vi "PDUS-SerialPortDataParse.vi"(9 "Numeric":i32, 10 "ErrorIntput":errorcluster, 11 "InputStr":string) -> (2 "ErrorOutput":errorcluster, 3 "OutputStr":string)   [LabVIEW 2023]
panel:
  out "TempNum":dbl=10.5556
  out "PressNum":dbl=10.5556
  out "Str":string
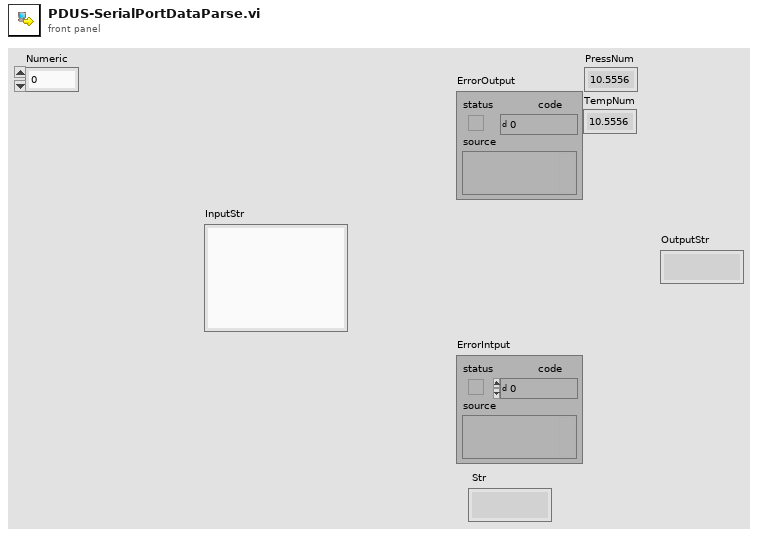
[diagram p1: front panel]
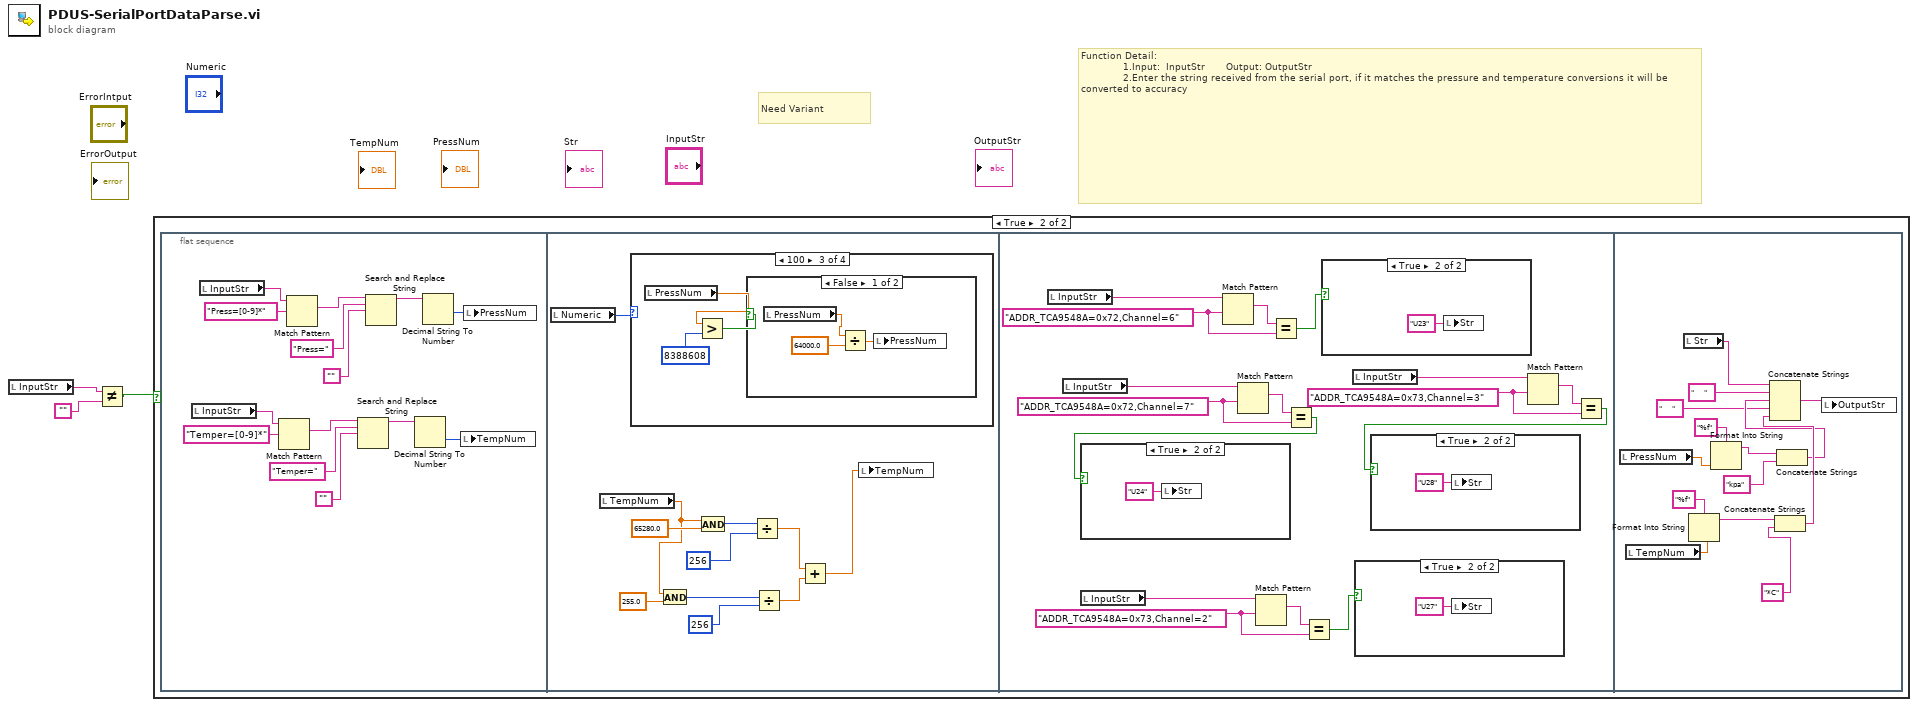
[diagram p0: block diagram]
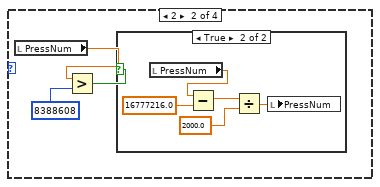
[diagram p4: hidden frame]
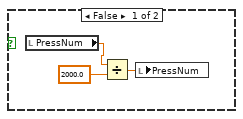
[diagram p5: hidden frame]
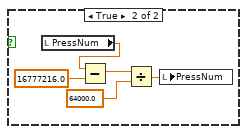
[diagram p6: hidden frame]
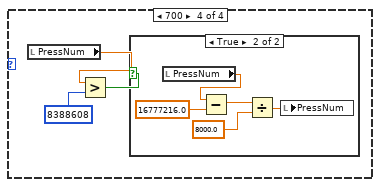
[diagram p7: hidden frame]
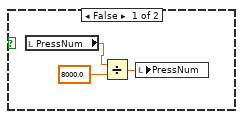
[diagram p8: hidden frame]
diagram:
  # "Function Detail:\n              1.Input:  InputStr       Output: OutputStr\n              2.Enter the string received from the serial port, if it matches the pressure and temperature conversions it will be converted to accuracy"
  # "Need Variant"
  n1 = local read "InputStr"() -> (w3:string)
  n2 = Not Equal?(x=w3, y="") -> (x != y?=w1:bool)
  n3 = case shown="True" w1 {
    frame False {
    }
    frame True {
      n4 = flat-sequence {
        frame #0 {
          n5 = local read "InputStr"() -> (w7:string)
          n6 = local read "InputStr"() -> (w16:string)
          n7 = Match Pattern(string=w7, regular expression="Temper=[0-9]*") -> (match substring=w8:string)  [unwired: 1 in, 3 out]
          n8 = Match Pattern(string=w16, regular expression="Press=[0-9]*") -> (match substring=w15:string)  [unwired: 1 in, 3 out]
          n9 = Search and Replace String(input string=w8, search string="Temper=", replace string="") -> (result string=w11:string)  [unwired: 5 in, 3 out]
          n10 = Search and Replace String(input string=w15, search string="Press=", replace string="") -> (result string=w12:string)  [unwired: 5 in, 3 out]
          n11 = Decimal String To Number(string=w11) -> (number=w4:i32)  [unwired: 2 in, 1 out]
          n12 = Decimal String To Number(string=w12) -> (number=w5:i32)  [unwired: 2 in, 1 out]
          n13 = local write "TempNum"(w4) -> ()
          n14 = local write "PressNum"(w5) -> ()
        }
        frame #1 {
          n15 = local read "Numeric"() -> (w28:i32)
          n16 = local read "TempNum"() -> (w22:dbl)
          n17 = case shown="100" w28 {
            frame 0, Default {
            }
            frame 2 {
              n18 = local read "PressNum"() -> (w30:dbl)
              n19 = Greater?(x=w30, y=8388608) -> (0:w31:bool)
              n20 = case shown="True" w31 {
                frame False {
                  n21 = local read "PressNum"() -> (w33:dbl)
                  n22 = Divide(x=w33, y=2000.0) -> (x/y=w34:dbl)
                  n23 = local write "PressNum"(w34) -> ()
                }
                frame True {
                  n24 = local read "PressNum"() -> (w39:dbl)
                  n25 = Subtract(x=w39, y=16777216.0) -> (x-y=w37:dbl)
                  n26 = Divide(x=w37, y=2000.0) -> (x/y=w35:dbl)
                  n27 = local write "PressNum"(w35) -> ()
                }
              }
            }
            frame 100 {
              n28 = local read "PressNum"() -> (w41:dbl)
              n29 = Greater?(x=w41, y=8388608) -> (0:w42:bool)
              n30 = case shown="False" w42 {
                frame False {
                  n31 = local read "PressNum"() -> (w44:dbl)
                  n32 = Divide(x=w44, y=64000.0) -> (x/y=w45:dbl)
                  n33 = local write "PressNum"(w45) -> ()
                }
                frame True {
                  n34 = local read "PressNum"() -> (w50:dbl)
                  n35 = Subtract(x=w50, y=16777216.0) -> (x-y=w48:dbl)
                  n36 = Divide(x=w48, y=64000.0) -> (x/y=w46:dbl)
                  n37 = local write "PressNum"(w46) -> ()
                }
              }
            }
            frame 700 {
              n38 = local read "PressNum"() -> (w52:dbl)
              n39 = Greater?(x=w52, y=8388608) -> (0:w53:bool)
              n40 = case shown="True" w53 {
                frame False {
                  n41 = local read "PressNum"() -> (w55:dbl)
                  n42 = Divide(x=w55, y=8000.0) -> (x/y=w56:dbl)
                  n43 = local write "PressNum"(w56) -> ()
                }
                frame True {
                  n44 = local read "PressNum"() -> (w61:dbl)
                  n45 = Subtract(x=w61, y=16777216.0) -> (x-y=w59:dbl)
                  n46 = Divide(x=w59, y=8000.0) -> (x/y=w57:dbl)
                  n47 = local write "PressNum"(w57) -> ()
                }
              }
            }
          }
          n48 = And(x=w22, y=255.0) -> (x .and. y?=w23:i32)
          n49 = And(x=w22, y=65280.0) -> (x .and. y?=w26:i32)
          n50 = Divide(x=w26, y=256) -> (x/y=w20:dbl)
          n51 = Divide(x=w23, y=256) -> (x/y=w19:dbl)
          n52 = Add(x=w20, y=w19) -> (x+y=w18:dbl)
          n53 = local write "TempNum"(w18) -> ()
        }
        frame #2 {
          w64 = "ADDR_TCA9548A=0x73,Channel=2" ("regular expression")
          w66 = "ADDR_TCA9548A=0x73,Channel=3" ("regular expression")
          w73 = "ADDR_TCA9548A=0x72,Channel=7" ("regular expression")
          w75 = "ADDR_TCA9548A=0x72,Channel=6" ("regular expression")
          n54 = local read "InputStr"() -> (w77:string)
          n55 = local read "InputStr"() -> (w71:string)
          n56 = local read "InputStr"() -> (w62:string)
          n57 = Match Pattern(string=w77, regular expression=w75) -> (match substring=w76:string)  [unwired: 1 in, 3 out]
          n58 = Match Pattern(string=w71, regular expression=w73) -> (match substring=w72:string)  [unwired: 1 in, 3 out]
          n59 = Match Pattern(string=w62, regular expression=w64) -> (match substring=w63:string)  [unwired: 1 in, 3 out]
          n60 = Equal?(x=w76, y=w75) -> (x = y?=w74:bool)
          n61 = Equal?(x=w72, y=w73) -> (x = y?=w70:bool)
          n62 = case shown="True" w70 {
            frame False {
            }
            frame True {
              n63 = local write "Str"("U24" ("Str")) -> ()
            }
          }
          n64 = Equal?(x=w63, y=w64) -> (x = y?=w65:bool)
          n65 = case shown="True" w74 {
            frame False {
            }
            frame True {
              n66 = local write "Str"("U23" ("Str")) -> ()
            }
          }
          n67 = local read "InputStr"() -> (w68:string)
          n68 = case shown="True" w65 {
            frame False {
            }
            frame True {
              n69 = local write "Str"("U27" ("Str")) -> ()
            }
          }
          n70 = Match Pattern(string=w68, regular expression=w66) -> (match substring=w67:string)  [unwired: 1 in, 3 out]
          n71 = Equal?(x=w67, y=w66) -> (x = y?=w69:bool)
          n72 = case shown="True" w69 {
            frame False {
            }
            frame True {
              n73 = local write "Str"("U28" ("Str")) -> ()
            }
          }
        }
        frame #3 {
          n74 = local read "PressNum"() -> (w86:dbl)
          n75 = local read "TempNum"() -> (w84:dbl)
          n76 = local read "Str"() -> (w88:string)
          n77 = Format Into String(format string="%f", w84) -> (resulting string=w82:string)  [unwired: 2 in, 1 out]
          n78 = Format Into String(format string="%f", w86) -> (resulting string=w85:string)  [unwired: 2 in, 1 out]
          n79 = Concatenate Strings(w82, "*C" ("string")) -> (w95:string)
          n80 = Concatenate Strings(w85, "kpa" ("string")) -> (w93:string)
          n81 = Concatenate Strings(w88, "     " ("string"), w93, "     " ("string"), w95) -> (w94:string)
          n82 = local write "OutputStr"(w94) -> ()
        }
      }
    }
  }
